vi "Create Command Packet 3_red.vi"(0 "Function #":u16, 1 "Camera ID (1)":u8=1, 3 "Acq. Mode/Type/Frame Mode/RO Mode":u8, 5 "Buffer/Avg #/Frames":u16, 7 "Exposure Time (ms)":u32, 9 "Camera Color":string(combo), 11 "Mode":u16, 12 "File Name":string, 13 "Paramater value":i32, 14 "Save As":u16(ring) items=["U16 FITS", "I16 FITS", "I32 FITS", "SGL FITS", "U16 TIFF", "I16 TIFF", "I32 TIFF", "SGL TIFF"], 15 "CCD Format Parameters":T1={"Serial Origin"=50, "Serial Length"=512, "Serial Binning"=1, "Parallel Origin"=0, "Parallel Length"=1024, "Parallel Binning"=1} {"Parallel Binning" min=1 max=5000 step=1; "Parallel Length" min=0 max=65535 step=1; "Parallel Origin" min=0 max=9000 step=1; "Serial Binning" min=1 max=5000 step=1; "Serial Length" min=0 max=65535 step=1; "Serial Origin" min=0 max=9000 step=1}) -> (6 "Cmd Packet":string)   [LabVIEW 2015]
uses:
  CCD Format.ctl
panel:
  # "Parallel"
  # "Serial"
  # "Origin"
  # "Length"
  # "Binning"
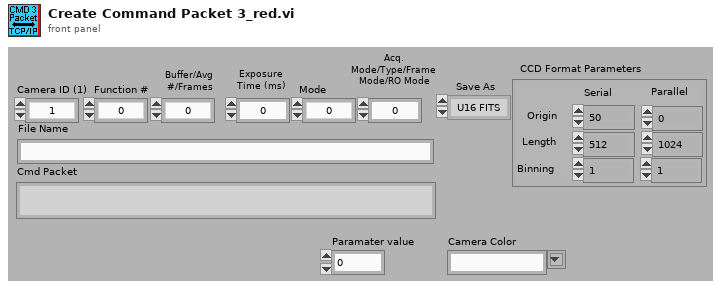
[diagram p1: front panel]
types:
  T1 = typedef "CCD Format.ctl" = cluster{"Serial Origin":i32, "Serial Length":i32, "Serial Binning":i32, "Parallel Origin":i32, "Parallel Length":i32, "Parallel Binning":i32}
  T2 = cluster{"Packet Length":u32, u8, "Camera ID (1)":u8, "Function #":u16, "Param Block Length":u16}
  T3 = cluster{u32, u8, "Camera ID (1)":u8, "Function #":u16, u16, "Exposure Time (ms)":u32, "Mode":u16, "Buffer/Avg #/Frames":u16, "Save As":u16}
  T4 = cluster{"Packet Length":u32, u8, "Camera ID (1)":u8, "Function #":u16, "Param Block Length":u16, "Buffer/Avg #/Frames":u16}
  T5 = cluster{u32, u8, "Camera ID (1)":u8, "Function #":u16, u16, "Save As":u16}
  T6 = cluster{"Packet Length":u32, u8, "Camera ID (1)":u8, "Function #":u16, "Param Block Length":u16, "Acq. Mode/Type/Frame Mode/RO Mode":u8}
  T7 = cluster{"Packet Length":u32, u8, "Camera ID (1)":u8, "Function #":u16, "Param Block Length":u16, dbl}
  T8 = cluster{"x":u32, u8, "Camera ID (1)":u8, "Function #":u16}
  T9 = cluster{"Packet Length":u32, u8, "Camera ID (1)":u8, "Function #":u16, "Param Block Length":u16, i32}
  T10 = cluster{"Packet Length":u32, u8, "Camera ID (1)":u8, "Function #":u16, "Param Block Length":u16, "CCD Format Parameters":T1}
  T11 = cluster{u32, u8, "Camera ID (1)":u8, "Function #":u16, u16, "Paramater value":i32}
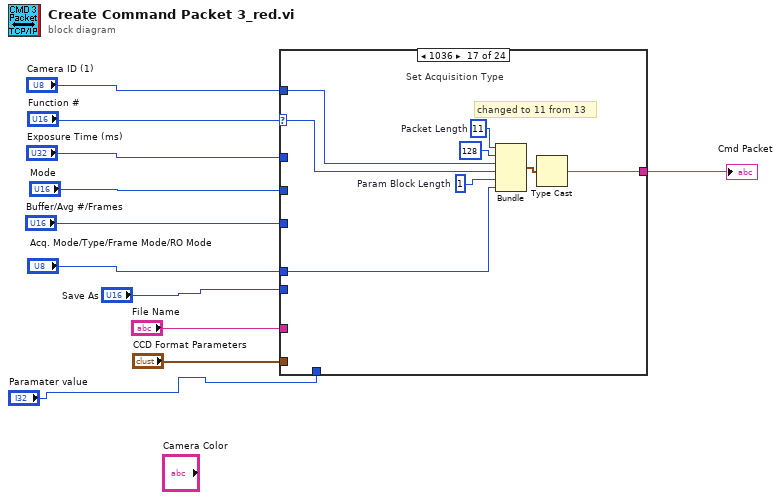
[diagram p0: block diagram]
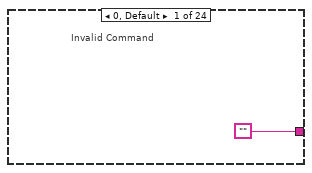
[diagram p2: hidden frame]
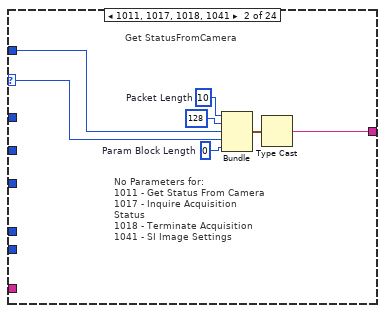
[diagram p3: hidden frame]
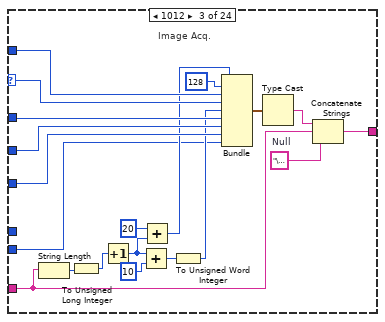
[diagram p4: hidden frame]
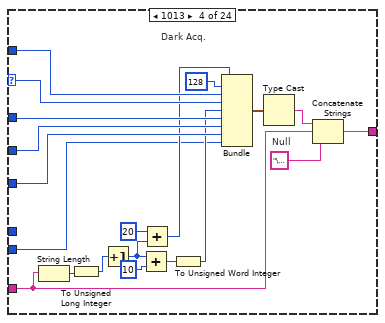
[diagram p5: hidden frame]
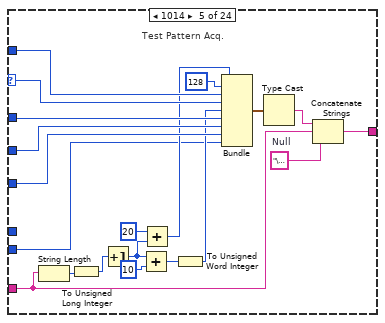
[diagram p6: hidden frame]
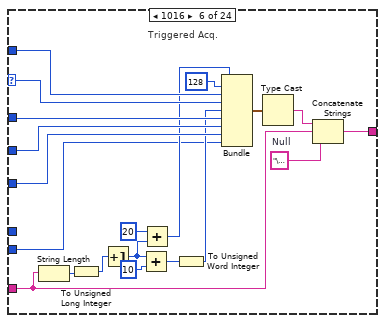
[diagram p7: hidden frame]
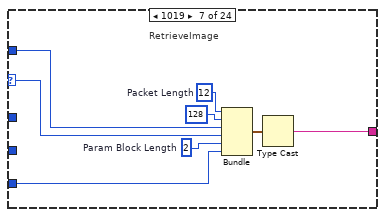
[diagram p8: hidden frame]
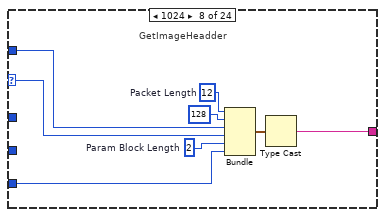
[diagram p9: hidden frame]
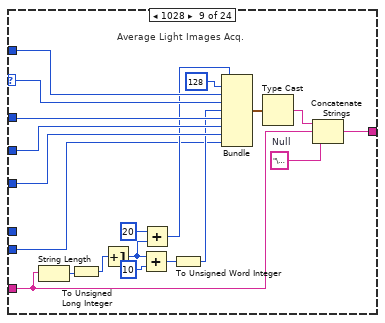
[diagram p10: hidden frame]
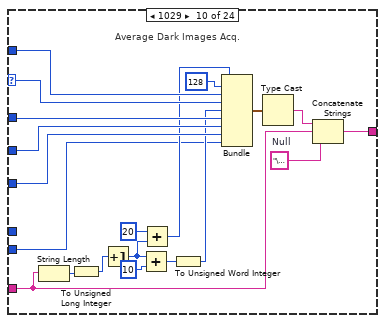
[diagram p11: hidden frame]
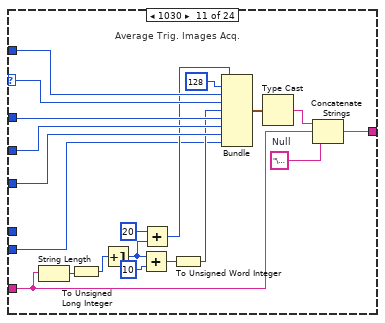
[diagram p12: hidden frame]
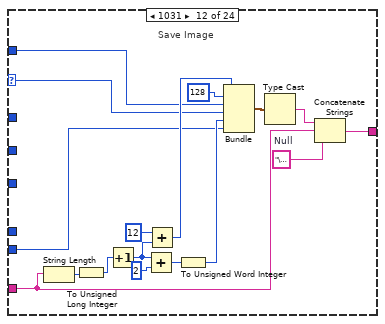
[diagram p13: hidden frame]
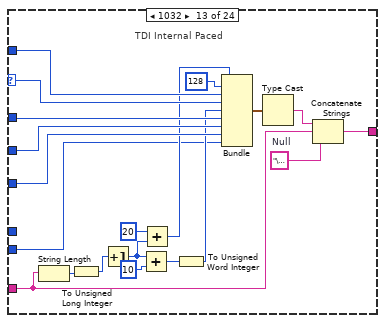
[diagram p14: hidden frame]
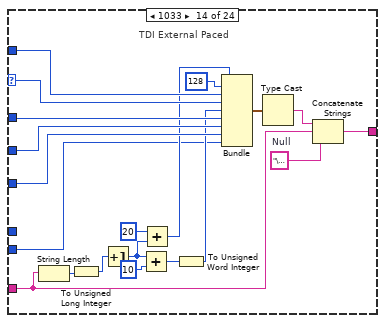
[diagram p15: hidden frame]
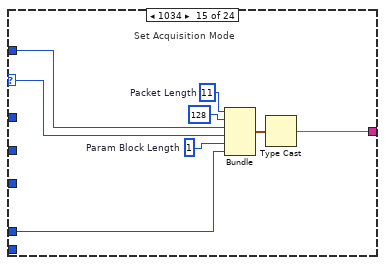
[diagram p16: hidden frame]
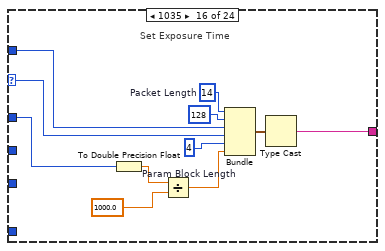
[diagram p17: hidden frame]
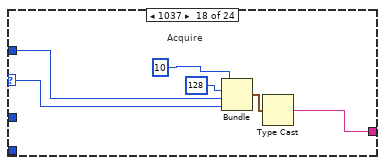
[diagram p18: hidden frame]
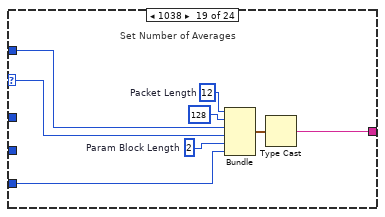
[diagram p19: hidden frame]
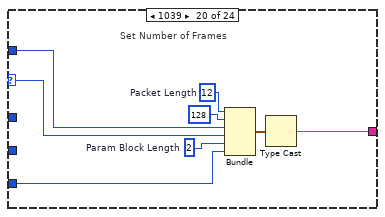
[diagram p20: hidden frame]
diagram:
  n1 = case shown="1036" "Function #" {
    selector: "Function #" -> [_ w16 w36 w56 w76 w96 w104 w110 w132 w152 w172 w177 w209 w229 w235 w246 w254 w262 w268 w276 w284 w293 w301 w320]
    tunnel: "Camera ID (1)" -> [_ w17 w37 w57 w77 w97 w105 w111 w133 w153 w173 w176 w210 w230 w236 w247 w255 w263 w269 w277 w285 w294 w302 w321]
    tunnel: "Exposure Time (ms)" -> [_ _ w35 w55 w75 w95 _ _ w131 w151 w171 _ w208 w228 _ w244 _ _ _ _ _ _ _ _]
    tunnel: "Mode" -> [_ _ w34 w54 w74 w94 _ _ w130 w150 w170 _ w207 w227 _ _ _ _ _ _ _ _ _ _]
    tunnel: "Buffer/Avg #/Frames" -> [_ _ w33 w53 w73 w93 w103 w109 w129 w149 w169 _ w206 w226 _ _ _ _ w266 w274 _ w292 _ _]
    tunnel: "File Name" -> [_ _ w24 w44 w64 w84 _ _ w120 w140 w160 w180 w197 w217 _ _ _ _ _ _ _ _ _ w313]
    tunnel: ["" w13 w22 w42 w62 w82 w100 w108 w118 w138 w158 w178 w195 w215 w234 w245 w253 w260 w267 w275 w283 w290 w300 w312] -> w2
    tunnel: "Save As" -> [_ _ w20 w40 w60 w80 _ _ w116 w136 w156 w179 w193 w213 _ _ _ _ _ _ _ _ _ _]
    tunnel: "Acq. Mode/Type/Frame Mode/RO Mode" -> [_ _ _ _ _ _ _ _ _ _ _ _ _ _ w233 _ w252 _ _ _ w282 _ _ _]
    tunnel: "CCD Format Parameters" -> [_ _ _ _ _ _ _ _ _ _ _ _ _ _ _ _ _ _ _ _ _ _ w299 _]
    tunnel: "Paramater value" -> [_ _ _ _ _ _ _ _ _ _ _ _ _ _ _ _ _ _ _ _ _ _ _ w319]
    frame 0, Default {
      # "Invalid Command"
    }
    frame 1011, 1017, 1018, 1041 {
      w14 = u16 0  # Param Block Length
      w15 = u32 10  # Packet Length
      # "No Parameters for:\n1011 - Get Status From Camera\n1017 - Inquire Acquisition Status\n1018 - Terminate Acquisition\n1041 - SI Image Settings"
      # "Get StatusFromCamera"
      n2 = Bundle("Packet Length"=w15, u8 128, "Camera ID (1)"=w17, "Function #"=w16, "Param Block Length"=w14) -> (w18:T2)  [unwired: 1 in]
      n3 = Type Cast(x=w18) -> (*(type *) &x=w13:string)  [unwired: 1 in]
    }
    frame 1012 {
      w23 = "\u0000"  # Null
      # "Image Acq."
      n4 = String Length(string=w24) -> (length=w32:i32)
      n5 = To Unsigned Long Integer(number=w32) -> (unsigned 32bit integer=w30:u32)
      n6 = Increment(x=w30) -> (x+1=w31:u32)
      n7 = Add(x=w31, y=u16 10) -> (x+y=w26:u32)
      n8 = Add(x=u16 20, y=w31) -> (x+y=w27:u32)
      n9 = To Unsigned Word Integer(number=w26) -> (unsigned 16bit integer=w21:u16)
      n10 = Bundle(w27, u8 128, "Camera ID (1)"=w37, "Function #"=w36, w21, "Exposure Time (ms)"=w35, "Mode"=w34, "Buffer/Avg #/Frames"=w33, "Save As"=w20) -> (w38:T3)  [unwired: 1 in]
      n11 = Type Cast(x=w38) -> (*(type *) &x=w25:string)  [unwired: 1 in]
      n12 = Concatenate Strings(w25, w24, w23) -> (w22:string)
    }
    frame 1013 {
      w43 = "\u0000"  # Null
      # "Dark Acq."
      n13 = String Length(string=w44) -> (length=w52:i32)
      n14 = To Unsigned Long Integer(number=w52) -> (unsigned 32bit integer=w50:u32)
      n15 = Increment(x=w50) -> (x+1=w51:u32)
      n16 = Add(x=w51, y=u16 10) -> (x+y=w46:u32)
      n17 = Add(x=u16 20, y=w51) -> (x+y=w47:u32)
      n18 = To Unsigned Word Integer(number=w46) -> (unsigned 16bit integer=w41:u16)
      n19 = Bundle(w47, u8 128, "Camera ID (1)"=w57, "Function #"=w56, w41, "Exposure Time (ms)"=w55, "Mode"=w54, "Buffer/Avg #/Frames"=w53, "Save As"=w40) -> (w58:T3)  [unwired: 1 in]
      n20 = Type Cast(x=w58) -> (*(type *) &x=w45:string)  [unwired: 1 in]
      n21 = Concatenate Strings(w45, w44, w43) -> (w42:string)
    }
    frame 1014 {
      w63 = "\u0000"  # Null
      # "Test Pattern Acq."
      n22 = String Length(string=w64) -> (length=w72:i32)
      n23 = To Unsigned Long Integer(number=w72) -> (unsigned 32bit integer=w70:u32)
      n24 = Increment(x=w70) -> (x+1=w71:u32)
      n25 = Add(x=w71, y=u16 10) -> (x+y=w66:u32)
      n26 = Add(x=u16 20, y=w71) -> (x+y=w67:u32)
      n27 = To Unsigned Word Integer(number=w66) -> (unsigned 16bit integer=w61:u16)
      n28 = Bundle(w67, u8 128, "Camera ID (1)"=w77, "Function #"=w76, w61, "Exposure Time (ms)"=w75, "Mode"=w74, "Buffer/Avg #/Frames"=w73, "Save As"=w60) -> (w78:T3)  [unwired: 1 in]
      n29 = Type Cast(x=w78) -> (*(type *) &x=w65:string)  [unwired: 1 in]
      n30 = Concatenate Strings(w65, w64, w63) -> (w62:string)
    }
    frame 1016 {
      w83 = "\u0000"  # Null
      # "Triggered Acq."
      n31 = String Length(string=w84) -> (length=w92:i32)
      n32 = To Unsigned Long Integer(number=w92) -> (unsigned 32bit integer=w90:u32)
      n33 = Increment(x=w90) -> (x+1=w91:u32)
      n34 = Add(x=w91, y=u16 10) -> (x+y=w86:u32)
      n35 = Add(x=u16 20, y=w91) -> (x+y=w87:u32)
      n36 = To Unsigned Word Integer(number=w86) -> (unsigned 16bit integer=w81:u16)
      n37 = Bundle(w87, u8 128, "Camera ID (1)"=w97, "Function #"=w96, w81, "Exposure Time (ms)"=w95, "Mode"=w94, "Buffer/Avg #/Frames"=w93, "Save As"=w80) -> (w98:T3)  [unwired: 1 in]
      n38 = Type Cast(x=w98) -> (*(type *) &x=w85:string)  [unwired: 1 in]
      n39 = Concatenate Strings(w85, w84, w83) -> (w82:string)
    }
    frame 1019 {
      w101 = u16 2  # Param Block Length
      w102 = u32 12  # Packet Length
      # "RetrieveImage"
      n40 = Bundle("Packet Length"=w102, u8 128, "Camera ID (1)"=w105, "Function #"=w104, "Param Block Length"=w101, "Buffer/Avg #/Frames"=w103) -> (w106:T4)  [unwired: 1 in]
      n41 = Type Cast(x=w106) -> (*(type *) &x=w100:string)  [unwired: 1 in]
    }
    frame 1024 {
      w112 = u16 2  # Param Block Length
      w113 = u32 12  # Packet Length
      # "GetImageHeadder"
      n42 = Bundle("Packet Length"=w113, u8 128, "Camera ID (1)"=w111, "Function #"=w110, "Param Block Length"=w112, "Buffer/Avg #/Frames"=w109) -> (w114:T4)  [unwired: 1 in]
      n43 = Type Cast(x=w114) -> (*(type *) &x=w108:string)  [unwired: 1 in]
    }
    frame 1028 {
      w119 = "\u0000"  # Null
      # "Average Light Images Acq."
      n44 = String Length(string=w120) -> (length=w128:i32)
      n45 = To Unsigned Long Integer(number=w128) -> (unsigned 32bit integer=w126:u32)
      n46 = Increment(x=w126) -> (x+1=w127:u32)
      n47 = Add(x=w127, y=u16 10) -> (x+y=w122:u32)
      n48 = Add(x=u16 20, y=w127) -> (x+y=w123:u32)
      n49 = To Unsigned Word Integer(number=w122) -> (unsigned 16bit integer=w117:u16)
      n50 = Bundle(w123, u8 128, "Camera ID (1)"=w133, "Function #"=w132, w117, "Exposure Time (ms)"=w131, "Mode"=w130, "Buffer/Avg #/Frames"=w129, "Save As"=w116) -> (w134:T3)  [unwired: 1 in]
      n51 = Type Cast(x=w134) -> (*(type *) &x=w121:string)  [unwired: 1 in]
      n52 = Concatenate Strings(w121, w120, w119) -> (w118:string)
    }
    frame 1029 {
      w139 = "\u0000"  # Null
      # "Average Dark Images Acq."
      n53 = String Length(string=w140) -> (length=w148:i32)
      n54 = To Unsigned Long Integer(number=w148) -> (unsigned 32bit integer=w146:u32)
      n55 = Increment(x=w146) -> (x+1=w147:u32)
      n56 = Add(x=w147, y=u16 10) -> (x+y=w142:u32)
      n57 = Add(x=u16 20, y=w147) -> (x+y=w143:u32)
      n58 = To Unsigned Word Integer(number=w142) -> (unsigned 16bit integer=w137:u16)
      n59 = Bundle(w143, u8 128, "Camera ID (1)"=w153, "Function #"=w152, w137, "Exposure Time (ms)"=w151, "Mode"=w150, "Buffer/Avg #/Frames"=w149, "Save As"=w136) -> (w154:T3)  [unwired: 1 in]
      n60 = Type Cast(x=w154) -> (*(type *) &x=w141:string)  [unwired: 1 in]
      n61 = Concatenate Strings(w141, w140, w139) -> (w138:string)
    }
    frame 1030 {
      w159 = "\u0000"  # Null
      # "Average Trig. Images Acq."
      n62 = String Length(string=w160) -> (length=w168:i32)
      n63 = To Unsigned Long Integer(number=w168) -> (unsigned 32bit integer=w166:u32)
      n64 = Increment(x=w166) -> (x+1=w167:u32)
      n65 = Add(x=w167, y=u16 10) -> (x+y=w162:u32)
      n66 = Add(x=u16 20, y=w167) -> (x+y=w163:u32)
      n67 = To Unsigned Word Integer(number=w162) -> (unsigned 16bit integer=w157:u16)
      n68 = Bundle(w163, u8 128, "Camera ID (1)"=w173, "Function #"=w172, w157, "Exposure Time (ms)"=w171, "Mode"=w170, "Buffer/Avg #/Frames"=w169, "Save As"=w156) -> (w174:T3)  [unwired: 1 in]
      n69 = Type Cast(x=w174) -> (*(type *) &x=w161:string)  [unwired: 1 in]
      n70 = Concatenate Strings(w161, w160, w159) -> (w158:string)
    }
    frame 1031 {
      w182 = "\u0000"  # Null
      # "Save Image"
      n71 = String Length(string=w180) -> (length=w190:i32)
      n72 = To Unsigned Long Integer(number=w190) -> (unsigned 32bit integer=w188:u32)
      n73 = Increment(x=w188) -> (x+1=w189:u32)
      n74 = Add(x=w189, y=u16 2) -> (x+y=w184:u32)
      n75 = Add(x=u16 12, y=w189) -> (x+y=w185:u32)
      n76 = To Unsigned Word Integer(number=w184) -> (unsigned 16bit integer=w181:u16)
      n77 = Bundle(w185, u8 128, "Camera ID (1)"=w176, "Function #"=w177, w181, "Save As"=w179) -> (w191:T5)  [unwired: 1 in]
      n78 = Type Cast(x=w191) -> (*(type *) &x=w183:string)  [unwired: 1 in]
      n79 = Concatenate Strings(w183, w180, w182) -> (w178:string)
    }
    frame 1032 {
      w196 = "\u0000"  # Null
      # "TDI Internal Paced"
      n80 = String Length(string=w197) -> (length=w205:i32)
      n81 = To Unsigned Long Integer(number=w205) -> (unsigned 32bit integer=w203:u32)
      n82 = Increment(x=w203) -> (x+1=w204:u32)
      n83 = Add(x=w204, y=u16 10) -> (x+y=w199:u32)
      n84 = Add(x=u16 20, y=w204) -> (x+y=w200:u32)
      n85 = To Unsigned Word Integer(number=w199) -> (unsigned 16bit integer=w194:u16)
      n86 = Bundle(w200, u8 128, "Camera ID (1)"=w210, "Function #"=w209, w194, "Exposure Time (ms)"=w208, "Mode"=w207, "Buffer/Avg #/Frames"=w206, "Save As"=w193) -> (w211:T3)  [unwired: 1 in]
      n87 = Type Cast(x=w211) -> (*(type *) &x=w198:string)  [unwired: 1 in]
      n88 = Concatenate Strings(w198, w197, w196) -> (w195:string)
    }
    frame 1033 {
      w216 = "\u0000"  # Null
      # "TDI External Paced"
      n89 = String Length(string=w217) -> (length=w225:i32)
      n90 = To Unsigned Long Integer(number=w225) -> (unsigned 32bit integer=w223:u32)
      n91 = Increment(x=w223) -> (x+1=w224:u32)
      n92 = Add(x=w224, y=u16 10) -> (x+y=w219:u32)
      n93 = Add(x=u16 20, y=w224) -> (x+y=w220:u32)
      n94 = To Unsigned Word Integer(number=w219) -> (unsigned 16bit integer=w214:u16)
      n95 = Bundle(w220, u8 128, "Camera ID (1)"=w230, "Function #"=w229, w214, "Exposure Time (ms)"=w228, "Mode"=w227, "Buffer/Avg #/Frames"=w226, "Save As"=w213) -> (w231:T3)  [unwired: 1 in]
      n96 = Type Cast(x=w231) -> (*(type *) &x=w218:string)  [unwired: 1 in]
      n97 = Concatenate Strings(w218, w217, w216) -> (w215:string)
    }
    frame 1034 {
      w237 = u16 1  # Param Block Length
      w238 = u32 11  # Packet Length
      # "Set Acquisition Mode"
      n98 = Bundle("Packet Length"=w238, u8 128, "Camera ID (1)"=w236, "Function #"=w235, "Param Block Length"=w237, "Acq. Mode/Type/Frame Mode/RO Mode"=w233) -> (w239:T6)  [unwired: 1 in]
      n99 = Type Cast(x=w239) -> (*(type *) &x=w234:string)  [unwired: 1 in]
    }
    frame 1035 {
      w248 = u16 4  # Param Block Length
      w249 = u32 14  # Packet Length
      # "Set Exposure Time"
      n100 = To Double Precision Float(number=w244) -> (double precision float=w243:dbl)
      n101 = Divide(x=w243, y=1000.0) -> (x/y=w242:dbl)
      n102 = Bundle("Packet Length"=w249, u8 128, "Camera ID (1)"=w247, "Function #"=w246, "Param Block Length"=w248, w242) -> (w250:T7)  [unwired: 1 in]
      n103 = Type Cast(x=w250) -> (*(type *) &x=w245:string)  [unwired: 1 in]
    }
    frame 1036 {
      w256 = u16 1  # Param Block Length
      w257 = u32 11  # Packet Length
      # "changed to 11 from 13"
      # "Set Acquisition Type"
      n104 = Bundle("Packet Length"=w257, u8 128, "Camera ID (1)"=w255, "Function #"=w254, "Param Block Length"=w256, "Acq. Mode/Type/Frame Mode/RO Mode"=w252) -> (w258:T6)  [unwired: 1 in]
      n105 = Type Cast(x=w258) -> (*(type *) &x=w253:string)  [unwired: 1 in]
    }
    frame 1037 {
      # "Acquire"
      n106 = Bundle("x"=u32 10, u8 128, "Camera ID (1)"=w263, "Function #"=w262) -> (w264:T8)  [unwired: 1 in]
      n107 = Type Cast(x=w264) -> (*(type *) &x=w260:string)  [unwired: 1 in]
    }
    frame 1038 {
      w270 = u16 2  # Param Block Length
      w271 = u32 12  # Packet Length
      # "Set Number of Averages"
      n108 = Bundle("Packet Length"=w271, u8 128, "Camera ID (1)"=w269, "Function #"=w268, "Param Block Length"=w270, "Buffer/Avg #/Frames"=w266) -> (w272:T4)  [unwired: 1 in]
      n109 = Type Cast(x=w272) -> (*(type *) &x=w267:string)  [unwired: 1 in]
    }
    frame 1039 {
      w278 = u16 2  # Param Block Length
      w279 = u32 12  # Packet Length
      # "Set Number of Frames"
      n110 = Bundle("Packet Length"=w279, u8 128, "Camera ID (1)"=w277, "Function #"=w276, "Param Block Length"=w278, "Buffer/Avg #/Frames"=w274) -> (w280:T4)  [unwired: 1 in]
      n111 = Type Cast(x=w280) -> (*(type *) &x=w275:string)  [unwired: 1 in]
    }
    frame 1042 {
      w286 = u16 1  # Param Block Length
      w287 = u32 11  # Packet Length
      # "Set Multi-Frame Acquisition Buffer Mode\nor Set RO Mode"
      n112 = Bundle("Packet Length"=w287, u8 128, "Camera ID (1)"=w285, "Function #"=w284, "Param Block Length"=w286, "Acq. Mode/Type/Frame Mode/RO Mode"=w282) -> (w288:T6)  [unwired: 1 in]
      n113 = Type Cast(x=w288) -> (*(type *) &x=w283:string)  [unwired: 1 in]
    }
    frame 1040 {
      w295 = u16 7  # Param Block Length
      w296 = u32 17  # Packet Length
      n114 = To Long Integer(number=w292) -> (32bit integer=w291:i32)
      n115 = Bundle("Packet Length"=w296, u8 128, "Camera ID (1)"=w294, "Function #"=w293, "Param Block Length"=w295, w291) -> (w297:T9)  [unwired: 1 in]
      n116 = Type Cast(x=w297) -> (*(type *) &x=w290:string)  [unwired: 1 in]
    }
    frame 1043 {
      w303 = u16 24  # Param Block Length
      w304 = u32 34  # Packet Length
      # "Set CCD Format"
      n117 = Bundle("Packet Length"=w304, u8 128, "Camera ID (1)"=w302, "Function #"=w301, "Param Block Length"=w303, "CCD Format Parameters"=w299) -> (w305:T10)  [unwired: 1 in]
      n118 = Type Cast(x=w305) -> (*(type *) &x=w300:string)  [unwired: 1 in]
    }
    frame 1044 {
      w315 = "\u0000"  # Null
      n119 = String Length(string=w313) -> (length=w318:i32)
      n120 = To Unsigned Long Integer(number=w318) -> (unsigned 32bit integer=w311:u32)
      n121 = Increment(x=w311) -> (x+1=w309:u32)
      n122 = Add(x=u16 14, y=w309) -> (x+y=w307:u32)
      n123 = Add(x=w309, y=u16 4) -> (x+y=w316:u32)
      n124 = To Unsigned Word Integer(number=w316) -> (unsigned 16bit integer=w308:u16)
      n125 = Bundle(w307, u8 128, "Camera ID (1)"=w321, "Function #"=w320, w308, "Paramater value"=w319) -> (w322:T11)  [unwired: 1 in]
      n126 = Type Cast(x=w322) -> (*(type *) &x=w314:string)  [unwired: 1 in]
      n127 = Concatenate Strings(w314, w313, w315) -> (w312:string)
    }
  }
  "Cmd Packet" <- w2
